vi "Create MC Cycle Engine Request Message Data .vi"(0 "Test Mode Enable?":bool, 2 "Cycle #":u8, 7 "MC Cycle Engine State":T1, 11 "Error In":errorcluster) -> (4 "MC Cycle Engine Request Message Data":string, 15 "Error Out":errorcluster)   [LabVIEW 2014]
doc: "This vi should be used to generate the Message Data for changing the MC Cycle Engine States."
uses:
  type defs/MC_Cycle_Engine_Request_State.ctl
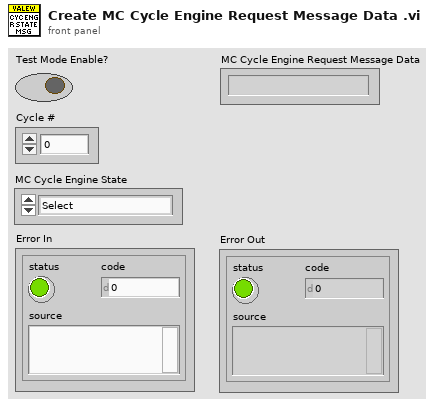
[diagram p1: front panel]
types:
  T1 = typedef "MC_Cycle_Engine_Request_State.ctl" = enum16{"Select", "Start", "Pause", "Resume", "Stop"}
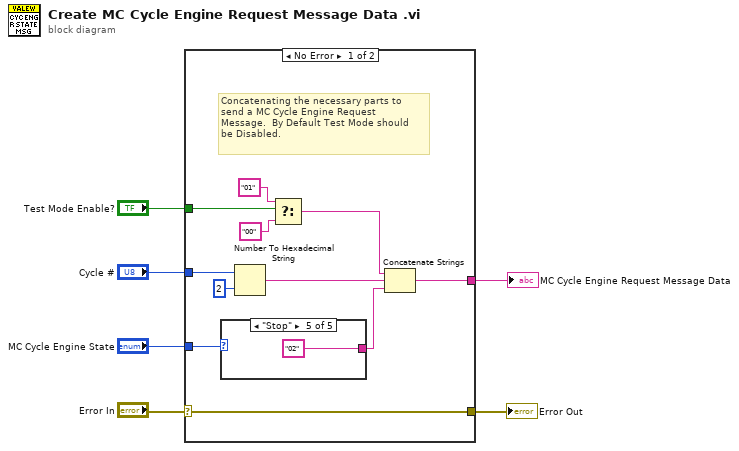
[diagram p0: block diagram]
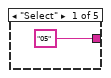
[diagram p2: hidden frame]
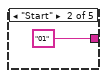
[diagram p3: hidden frame]
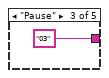
[diagram p4: hidden frame]
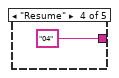
[diagram p5: hidden frame]
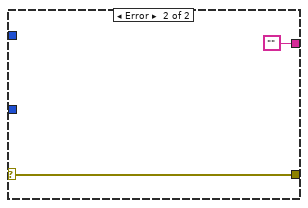
[diagram p6: hidden frame]
diagram:
  n1 = case shown="No Error" "Error In" {
    selector: "Error In" -> [w16 w23]
    tunnel: "Test Mode Enable?" -> [w13 _]
    tunnel: "MC Cycle Engine State" -> [w17 _]
    tunnel: [w16 w23] -> w4
    tunnel: "Cycle #" -> [w15 _]
    tunnel: [w7 ""] -> w1
    frame No Error {
      # "Concatenating the necessary parts to\nsend a MC Cycle Engine Request \nMessage.  By Default Test Mode should\nbe Disabled."
      n2 = case shown="\"Stop\"" w17 {
        tunnel: ["05" ("Message") "01" ("Message") "03" ("Message") "04" ("Message") "02" ("Message")] -> w8
        frame "Select" {
        }
        frame "Start" {
        }
        frame "Pause" {
        }
        frame "Resume" {
        }
        frame "Stop" {
        }
      }
      n3 = Number To Hexadecimal String(1:i16 2 ("width (-)"), 2:w15) -> (0:w9:string)
      n4 = Select(t="01" ("Message"), s=w13, f="00" ("Message")) -> (s? t:f=w10:string)
      n5 = Concatenate Strings(w10, w9, w8) -> (w7:string)
    }
    frame Error {
    }
  }
  "Error Out" <- w4
  "MC Cycle Engine Request Message Data" <- w1
